vi "parse_Odometry.vi"(0 "msg in":string, 3 "error in":errorcluster) -> (5 "Odometry":T1, 6 "msg out":string, 7 "Header":T2, 8 "child_frame_id":string, 9 "error out":errorcluster)   [LabVIEW 2016]
doc: "Parses a message into an odometry"
uses:
  std_msgs/subs/parse_string_scalar.vi
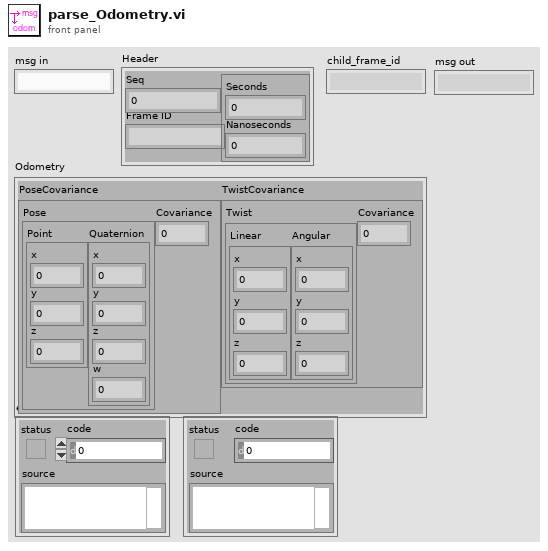
[diagram p1: front panel]
types:
  T1 = cluster{"PoseCovariance":cluster{"Pose":cluster{"Point":cluster{"x":dbl, "y":dbl, "z":dbl}, "Quaternion":cluster{"x":dbl, "y":dbl, "z":dbl, "w":dbl}}, "Covariance":dbl}, "TwistCovariance":cluster{"Twist":cluster{"Linear":cluster{"x":dbl, "y":dbl, "z":dbl}, "Angular":cluster{"x":dbl, "y":dbl, "z":dbl}}, "Covariance":dbl}}
  T2 = cluster{"Seq":u32, "Frame ID":string, "Timestamp":cluster{"Seconds":i32, "Nanoseconds":i32}}
  T3 = cluster{"Pose":cluster{"Point":cluster{"x":dbl, "y":dbl, "z":dbl}, "Quaternion":cluster{"x":dbl, "y":dbl, "z":dbl, "w":dbl}}, "Covariance":dbl}
  T4 = cluster{"Twist":cluster{"Linear":cluster{"x":dbl, "y":dbl, "z":dbl}, "Angular":cluster{"x":dbl, "y":dbl, "z":dbl}}, "Covariance":dbl}
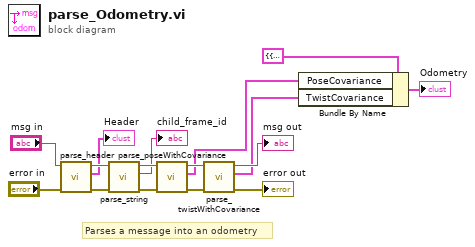
[diagram p0: block diagram]
diagram:
  # "Parses a message into an odometry"
  n1 = call "parse_header.vi"("error in"="error in", "msg in"="msg in") -> ("error out"=w11:errorcluster, "Header"=→"Header":T2, "msg out"=w15:string)  [unwired: 3 in]
  n2 = call-poly "parse_string.vi"("error in"=w11, "msg in"=w15) -> ("error out"=w12:errorcluster, "string"=→"child_frame_id":string, "msg out"=w7:string)  [unwired: 3 in]
  n3 = call "parse_poseWithCovariance.vi"("error in (no error)"=w12, "msg in"=w7) -> ("error out"=w14:errorcluster, "PoseCovariance"=w3:T3, "msg out"=w13:string)  [unwired: 3 in]
  n4 = call "parse_twistWithCovariance.vi"("error in"=w14, "msg in"=w13) -> ("error out"=→"error out":errorcluster, "TwistCovariance"=w2:T4, "msg out"=→"msg out":string)  [unwired: 3 in]
  n5 = Bundle By Name(cluster=T1 {"PoseCovariance"={"Pose"={"Point"={"x"=0.0, "y"=0.0, "z"=0.0}, "Quaternion"={"x"=0.0, "y"=0.0, "z"=0.0, "w"=0.0}}, "Covariance"=0.0}, "TwistCovariance"={"Twist"={"Linear"={"x"=0.0, "y"=0.0, "z"=0.0}, "Angular"={"x"=0.0, "y"=0.0, "z"=0.0}}, "Covariance"=0.0}} ("Odometry"), "PoseCovariance"=w3, "TwistCovariance"=w2) -> (→"Odometry":T1)
